vi "20220112 sub 1 ABC put select-1.vi"(0 "ABC":i32) -> (2 "ABC path out go catch":cluster{"X":dbl, "Y":dbl}[](array[cluster]))   [LabVIEW 2019]
uses:
  subVI/move/move array.ctl
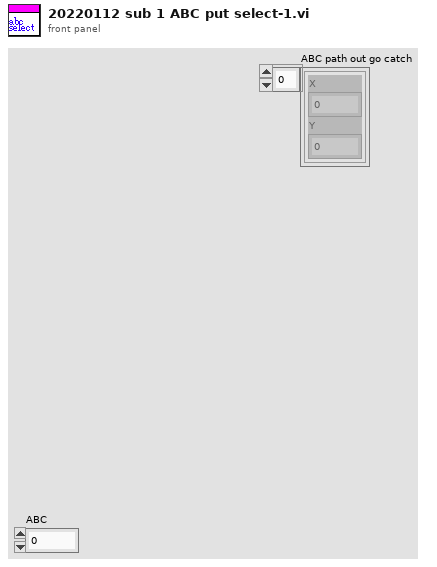
[diagram p1: front panel]
types:
  T1 = typedef "move array.ctl" = cluster{"X":dbl, "Y":dbl}[]
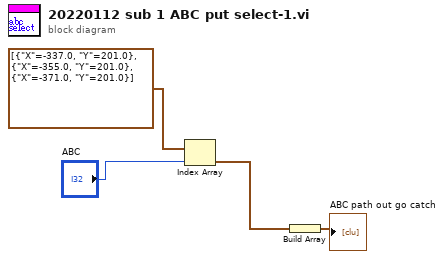
[diagram p0: block diagram]
diagram:
  n1 = Index Array(array=T1 [{"X"=-337.0, "Y"=201.0}, {"X"=-355.0, "Y"=201.0}, {"X"=-371.0, "Y"=201.0}] ("Array"), index="ABC") -> (element=w2:cluster{"X":dbl, "Y":dbl})
  n2 = Build Array(w2) -> (→"ABC path out go catch":cluster{"X":dbl, "Y":dbl}[])
